vi "S2C_ManageMenu.vi"(8 "Error In":errorcluster, 10 "ItemPath":string, 11 "Q-Ref":refnum<queue>) -> (0 "Error Out":errorcluster)   [LabVIEW 2015]
doc: "Manages the user runtime menu selections."
uses:
  Globals/S2C_GlobalMenus.vi
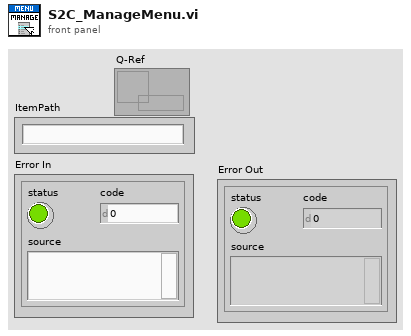
[diagram p1: front panel]
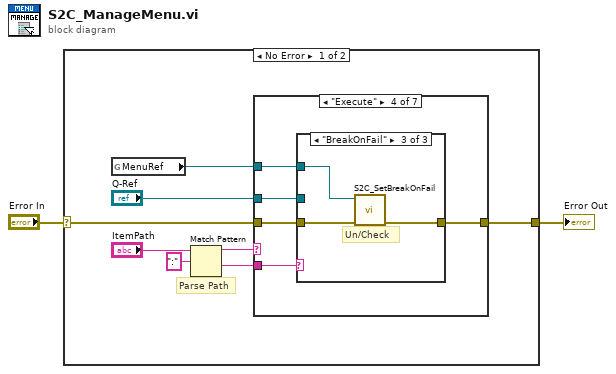
[diagram p0: block diagram]
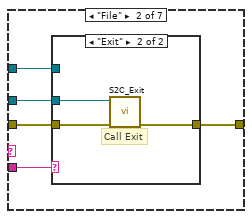
[diagram p3: hidden frame]
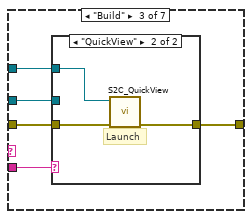
[diagram p5: hidden frame]
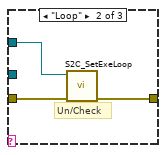
[diagram p8: hidden frame]
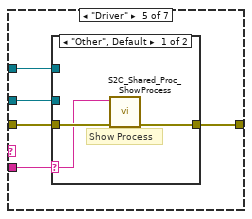
[diagram p9: hidden frame]
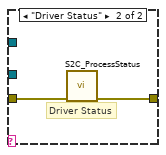
[diagram p10: hidden frame]
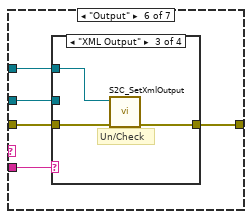
[diagram p11: hidden frame]
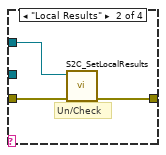
[diagram p13: hidden frame]
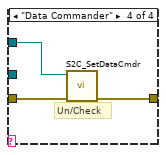
[diagram p14: hidden frame]
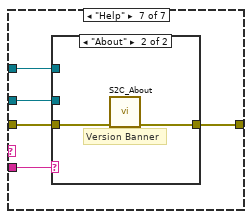
[diagram p15: hidden frame]
diagram:
  n1 = case shown="No Error" "Error In" {
    selector: "Error In" -> [w7 w75]
    tunnel: [w6 w75] -> w1
    frame No Error {
      # "Parse Path"
      n2 = global read "S2C_GlobalMenus.vi" "MenuRef"() -> (w3:refnum<k9>)
      n3 = Match Pattern(string="ItemPath", regular expression=":") -> (before substring=w9:string, after substring=w8:string)  [unwired: 1 in, 2 out]
      n4 = case shown="\"Execute\"" w9 {
        tunnel: w7 -> [w11 w15 w24 w33 w45 w55 w70]
        tunnel: w8 -> [_ w16 w25 w34 w46 w56 w71]
        tunnel: [w11 w14 w23 w32 w44 w54 w69] -> w6
        tunnel: "Q-Ref" -> [_ w13 w22 w31 w43 w53 w68]
        tunnel: w3 -> [_ w12 w21 w30 w42 w52 w67]
        frame "Other", Default {
        }
        frame "File" {
          n5 = case shown="\"Exit\"" w16 {
            tunnel: w15 -> [w17 w20]
            tunnel: [w17 w18] -> w14
            tunnel: w13 -> [_ w19]
            tunnel: w12 -> [_ _]
            frame "Other", Default {
            }
            frame "Exit" {
              # "Call Exit"
              n6 = call "S2C_Exit.vi"("Error In"=w20, "S2C-Q"=w19) -> ("Error Out"=w18:errorcluster)  [unwired: 8 in, 1 out]
            }
          }
        }
        frame "Build" {
          n7 = case shown="\"QuickView\"" w25 {
            tunnel: w24 -> [w26 w29]
            tunnel: [w26 w28] -> w23
            tunnel: w22 -> [_ _]
            tunnel: w21 -> [_ w27]
            frame "Other", Default {
            }
            frame "QuickView" {
              # "Launch"
              n8 = call "S2C_QuickView.vi"("Error In"=w29, "MenuRef"=w27) -> ("Error Out"=w28:errorcluster)  [unwired: 9 in]
            }
          }
        }
        frame "Execute" {
          n9 = case shown="\"BreakOnFail\"" w34 {
            tunnel: w33 -> [w35 w38 w41]
            tunnel: [w35 w37 w40] -> w32
            tunnel: w31 -> [_ _ _]
            tunnel: w30 -> [_ w36 w39]
            frame "Other", Default {
            }
            frame "Loop" {
              # "Un/Check"
              n10 = call "S2C_SetExeLoop.vi"("Error In"=w38, "MenuRef"=w36) -> ("Error Out"=w37:errorcluster)  [unwired: 9 in]
            }
            frame "BreakOnFail" {
              # "Un/Check"
              n11 = call "S2C_SetBreakOnFail.vi"("Error In"=w41, "MenuRef"=w39) -> ("Error Out"=w40:errorcluster)  [unwired: 9 in]
            }
          }
        }
        frame "Driver" {
          n12 = case shown="\"Other\", Default" w46 {
            selector: w46 -> [w47 _]
            tunnel: w45 -> [w49 w51]
            tunnel: [w48 w50] -> w44
            tunnel: w43 -> [_ _]
            tunnel: w42 -> [_ _]
            frame "Other", Default {
              # "Show Process"
              n13 = call "S2C_Shared_Proc_ShowProcess.vi"("Error In"=w49, "ProcessName"=w47) -> ("Error Out"=w48:errorcluster)  [unwired: 9 in]
            }
            frame "Driver Status" {
              # "Driver Status"
              n14 = call "S2C_ProcessStatus.vi"("Error In"=w51) -> ("Error Out"=w50:errorcluster)  [unwired: 10 in]
            }
          }
        }
        frame "Output" {
          n15 = case shown="\"XML Output\"" w56 {
            tunnel: w55 -> [w57 w60 w63 w66]
            tunnel: [w57 w59 w62 w65] -> w54
            tunnel: w53 -> [_ _ _ _]
            tunnel: w52 -> [_ w58 w61 w64]
            frame "Other", Default {
            }
            frame "Local Results" {
              # "Un/Check"
              n16 = call "S2C_SetLocalResults.vi"("Error In"=w60, "MenuRef"=w58) -> ("Error Out"=w59:errorcluster)  [unwired: 9 in]
            }
            frame "XML Output" {
              # "Un/Check"
              n17 = call "S2C_SetXmlOutput.vi"("Error In"=w63, "MenuRef"=w61) -> ("Error Out"=w62:errorcluster)  [unwired: 9 in]
            }
            frame "Data Commander" {
              # "Un/Check"
              n18 = call "S2C_SetDataCmdr.vi"("Error In"=w66, "MenuRef"=w64) -> ("Error Out"=w65:errorcluster)  [unwired: 9 in]
            }
          }
        }
        frame "Help" {
          n19 = case shown="\"About\"" w71 {
            tunnel: w70 -> [w72 w74]
            tunnel: [w72 w73] -> w69
            tunnel: w68 -> [_ _]
            tunnel: w67 -> [_ _]
            frame "Other", Default {
            }
            frame "About" {
              # "Version Banner"
              n20 = call "S2C_About.vi"("Error In"=w74) -> ("Error Out"=w73:errorcluster)  [unwired: 10 in]
            }
          }
        }
      }
    }
    frame Error {
    }
  }
  "Error Out" <- w1
